vi "OTrig_l.vi"(8 "error in (no error)":errorcluster, 11 "drv":u32) -> (0 "error out":errorcluster)   [LabVIEW 2015, in "ESLSCDLL.lvlib"]
uses:
  ESLSCDLL.lvlib
  ESLSCDLL.dll
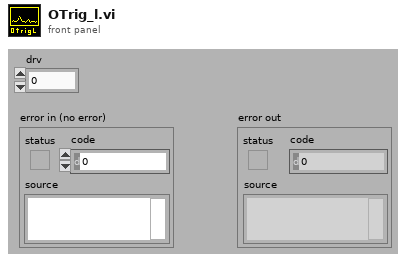
[diagram p1: front panel]
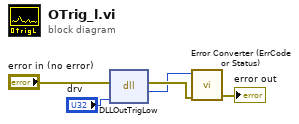
[diagram p0: block diagram]
diagram:
  n1 = dll-call lib="C:/Users/flori/Nextcloud/Dokumente/Stresing/Windows/lv64/board.vis/ESLSCDLL.dll" fn="DLLOutTrigLow"(error in="error in (no error)", "drv"="drv") -> (error out=w2:errorcluster, "es_status_codes"=w1:i32)  [unwired: 3 in, 1 out]
  n2 = call "Error Converter (ErrCode or Status).vi"("error in (no error)"=w2, "error code"=w1) -> ("error out"=→"error out":errorcluster)  [unwired: 9 in]
